vi "Close.vi"(8 "error in":errorcluster, 11 "Resistance Control in":refnum<class "Resistance Control.lvclass">) -> (0 "error out":errorcluster, 3 "Resistance Control out":refnum<class "Resistance Control.lvclass">)   [LabVIEW 2023, in "Resistance Control.lvclass"]
uses:
  Resistance Control.lvclass
  Resistance Control.lvclass/Resistance Control.ctl
  <vilib>/ADAS Replay HIL/AdasHilServices/AdasHilChannelServices.lvlib
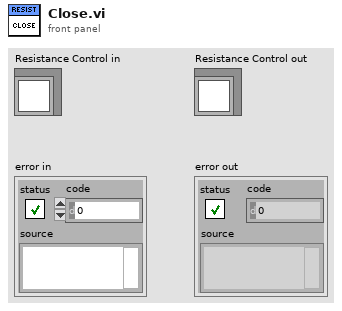
[diagram p1: front panel]
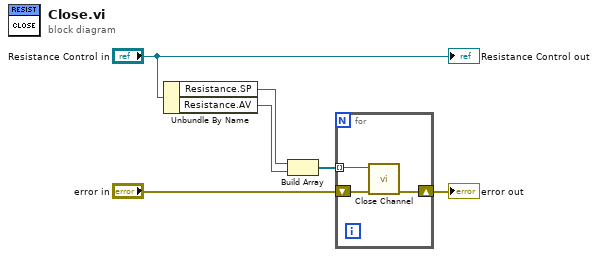
[diagram p0: block diagram]
diagram:
  n1 = Unbundle By Name("Resistance Control in") -> ("Resistance.SP"=w3:refnum<k21>, "Resistance.AV"=w4:refnum<k21>)
  n2 = Build Array(w3, w4) -> (w1:refnum<k21>[])
  n3 = for {
    shift-right: [w9] -> w6
    shift-left: "error in" -> [w8]
    tunnel: w1 -> [w7] mode=indexing
    n4 = call <vilib>:"Close Channel.vi"("error in"=w8, "ADAS HIL Channel"=w7) -> ("error out"=w9:errorcluster)  [unwired: 9 in]
  }
  "error out" <- w6
  "Resistance Control out" <- "Resistance Control in"
